vi "Write.vi"(7 "nonFull":refnum<k4>, 8 "element in":T3, 10 "parms in":T2={"subchannel"=0, "size (0)"=0, "abort (F)"=FALSE, "timeout"=-1, "ack id (0)"=0, "last elt? (F)"=FALSE, "valid? (T)"=FALSE, "GUID"=""}, 11 "MessengerMCPU in":refnum<class "MessengerMCPU.lvclass">) -> (0 "element out":T3, 1 "wait":bool, 2 "parms out":T1, 3 "MessengerMCPU out":refnum<class "MessengerMCPU.lvclass">)   [LabVIEW 2019, in "MessengerM.lvlib" / "MessengerMCPU.lvclass"]
uses:
  MessengerMCPU.lvclass
  ParmsOut.ctl
  MessengerM.lvlib
  SubChannelCPU/SubChannelCPU.lvclass
  Element.ctl
  ParmsIn.ctl
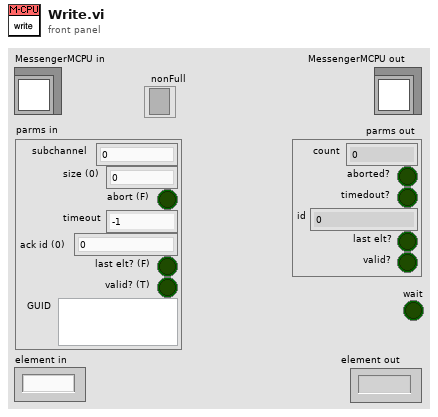
[diagram p1: front panel]
types:
  T1 = typedef "MessengerM.lvlib/ParmsOut.ctl" = cluster{"count":i32, "aborted?":bool, "timedout?":bool, "id":u32, "last elt?":bool, "valid?":bool}
  T2 = typedef "MessengerM.lvlib/ParmsIn.ctl" = cluster{"subchannel":i32, "size (0)":i32, "abort (F)":bool, "timeout":i32, "ack id (0)":u32, "last elt? (F)":bool, "valid? (T)":bool, "GUID":string}
  T3 = typedef "MessengerM.lvlib/Element.ctl" = string
  T4 = cluster{"GUID":string, "sub":refnum<class "SubChannelCPU.lvclass">}[]
  T5 = cluster{"GUID":string, "sub":refnum<class "SubChannelCPU.lvclass">}
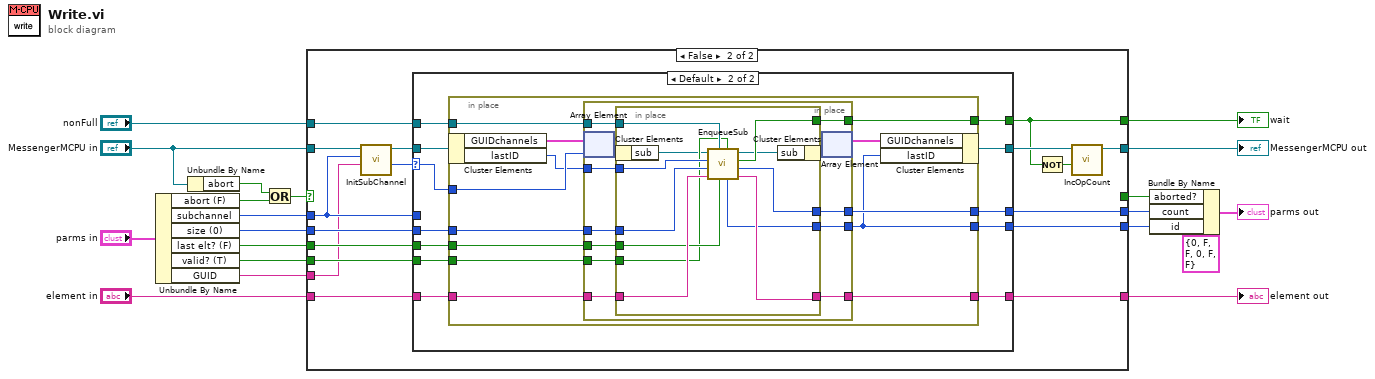
[diagram p0: block diagram]
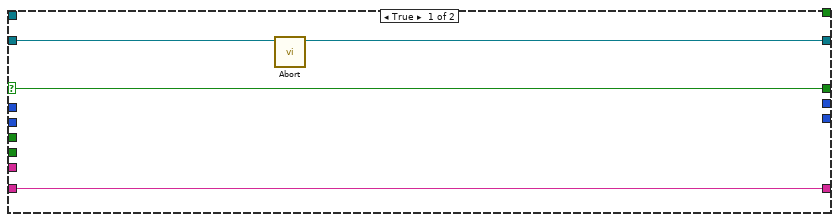
[diagram p2: hidden frame]
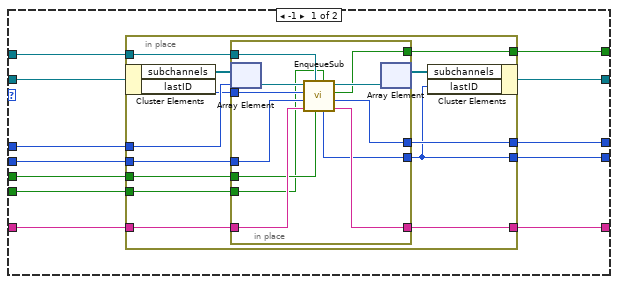
[diagram p3: hidden frame]
diagram:
  n1 = Unbundle By Name("parms in") -> ("abort (F)"=w9:bool, "subchannel"=w11:i32, "size (0)"=w10:i32, "last elt? (F)"=w3:bool, "valid? (T)"=w2:bool, "GUID"=w1:string)
  n2 = Unbundle By Name("MessengerMCPU in") -> ("abort"=w20:bool)
  n3 = Or(x=w20, y=w9) -> (x .or. y?=w19:bool)
  n4 = case shown="False" w19 {
    selector: w19 -> [w23 _]
    tunnel: [w21 w28] -> w16
    tunnel: [_ w41] -> w6
    tunnel: [w23 _] -> w4
    tunnel: [w24 w40] -> w17
    tunnel: [_ w27] -> w15
    tunnel: "element in" -> [w24 w39]
    tunnel: "MessengerMCPU in" -> [w22 w34]
    tunnel: [_ w38] -> w5
    tunnel: w11 -> [_ w33]
    tunnel: w10 -> [_ w37]
    tunnel: "nonFull" -> [_ w36]
    tunnel: w3 -> [_ w35]
    tunnel: w2 -> [_ w31]
    tunnel: w1 -> [_ w26]
    frame True {
      n5 = call-dynamic "Abort.vi"("MessengerMCPU in"=w22) -> ("MessengerMCPU out"=w21:refnum<class "MessengerMCPU.lvclass">)  [unwired: 10 in]
    }
    frame False {
      n6 = call "InitSubChannel.vi"("GUID"=w26, "subchannel"=w33, "MessengerMCPU in"=w34) -> ("GUIDsubchannel"=w25:i32, "MessengerMCPU out"=w32:refnum<class "MessengerMCPU.lvclass">)  [unwired: 7 in]
      n7 = case shown="Default" w25 {
        selector: w25 -> [_ w79]
        tunnel: [w53 w90] -> w41
        tunnel: [w52 w89] -> w40
        tunnel: w39 -> [w51 w88]
        tunnel: [w50 w87] -> w38
        tunnel: w37 -> [w49 w86]
        tunnel: w36 -> [w48 w85]
        tunnel: w35 -> [w47 w84]
        tunnel: w33 -> [w46 _]
        tunnel: w32 -> [w45 w83]
        tunnel: w31 -> [w44 w82]
        tunnel: [w43 w81] -> w29
        tunnel: [w42 w80] -> w27
        frame -1 {
          n8 = in-place {
            in-place-border: [w66] -> w53
            in-place-border: [w65] -> w52
            in-place-border: w51 -> [w64]
            in-place-border: [w58] -> w50
            in-place-border: [w63] -> w42
            in-place-border: w46 -> [w60]
            in-place-border: w49 -> [w59]
            in-place-border: w48 -> [w56]
            in-place-border: w47 -> [w55]
            in-place-border: w44 -> [w54]
            n9 = in-place-cluster #1(w45) -> ("subchannels"=w62:refnum<class "SubChannelCPU.lvclass">[], "lastID"=w57:u32)
            n10 = in-place {
              in-place-border: [w71] -> w66
              in-place-border: [w78] -> w65
              in-place-border: w64 -> [w74]
              in-place-border: [w70] -> w58
              in-place-border: [w72] -> w63
              in-place-border: w59 -> [w75]
              in-place-border: w57 -> [w73]
              in-place-border: w56 -> [w69]
              in-place-border: w55 -> [w68]
              in-place-border: w54 -> [w67]
              n11 = in-place-array #2(w62, w60) -> (w76:refnum<class "SubChannelCPU.lvclass">)
              n12 = call-dynamic "EnqueueSub.vi"("is valid (T)"=w67, "is last element (F)"=w68, "nonFull"=w69, "element in"=w74, "size"=w75, "lastID"=w73, "SubChannel in"=w76) -> ("element out"=w78:T3, "count"=w71:i32, "wait"=w72:bool, "SubChannel out"=w77:refnum<class "SubChannelCPU.lvclass">, "id"=w70:u32)
              n13 = in-place-array #2(w77) -> (w61:refnum<class "SubChannelCPU.lvclass">[])  [unwired: 1 out]
            }
            n14 = in-place-cluster #1("subchannels"=w61, "lastID"=w58) -> (w43:refnum<class "MessengerMCPU.lvclass">)
          }
        }
        frame Default {
          n15 = in-place {
            in-place-border: [w103] -> w90
            in-place-border: [w102] -> w89
            in-place-border: w88 -> [w101]
            in-place-border: [w95] -> w87
            in-place-border: [w100] -> w80
            in-place-border: w79 -> [w97]
            in-place-border: w86 -> [w96]
            in-place-border: w85 -> [w93]
            in-place-border: w84 -> [w92]
            in-place-border: w82 -> [w91]
            n16 = in-place-cluster #3(w83) -> ("GUIDchannels"=w99:T4, "lastID"=w94:u32)
            n17 = in-place {
              in-place-border: [w110] -> w103
              in-place-border: [w115] -> w102
              in-place-border: w101 -> [w113]
              in-place-border: [w109] -> w95
              in-place-border: [w111] -> w100
              in-place-border: w96 -> [w114]
              in-place-border: w94 -> [w112]
              in-place-border: w93 -> [w108]
              in-place-border: w92 -> [w107]
              in-place-border: w91 -> [w106]
              n18 = in-place-array #4(w99, w97) -> (w105:T5)
              n19 = in-place {
                in-place-border: [w127] -> w115
                in-place-border: w114 -> [w126]
                in-place-border: w113 -> [w125]
                in-place-border: w112 -> [w124]
                in-place-border: [w123] -> w111
                in-place-border: [w122] -> w110
                in-place-border: [w121] -> w109
                in-place-border: w108 -> [w120]
                in-place-border: w107 -> [w119]
                in-place-border: w106 -> [w118]
                n20 = in-place-cluster #5(w105) -> ("sub"=w117:refnum<class "SubChannelCPU.lvclass">)
                n21 = call-dynamic "EnqueueSub.vi"("is valid (T)"=w118, "is last element (F)"=w119, "nonFull"=w120, "element in"=w125, "size"=w126, "lastID"=w124, "SubChannel in"=w117) -> ("element out"=w127:T3, "count"=w122:i32, "wait"=w123:bool, "SubChannel out"=w116:refnum<class "SubChannelCPU.lvclass">, "id"=w121:u32)
                n22 = in-place-cluster #5("sub"=w116) -> (w104:T5)
              }
              n23 = in-place-array #4(w104) -> (w98:T4)  [unwired: 1 out]
            }
            n24 = in-place-cluster #3("GUIDchannels"=w98, "lastID"=w95) -> (w81:refnum<class "MessengerMCPU.lvclass">)
          }
        }
      }
      n25 = Not(x=w27) -> (.not. x?=w30:bool)
      n26 = call-dynamic "IncOpCount.vi"("inc?"=w30, "MessengerMCPU in"=w29) -> ("MessengerMCPU out"=w28:refnum<class "MessengerMCPU.lvclass">)  [unwired: 9 in]
    }
  }
  "MessengerMCPU out" <- w16
  "element out" <- w17
  "wait" <- w15
  n27 = Bundle By Name(cluster=T1 {"count"=0, "aborted?"=FALSE, "timedout?"=FALSE, "id"=0, "last elt?"=FALSE, "valid?"=FALSE} ("parms out"), "aborted?"=w4, "count"=w6, "id"=w5) -> (→"parms out":T1)
